vi "HexapodAcquireHardware.vi"(8 "error in (no error)":errorcluster, 11 "C-887 in":refnum<class "C-887.lvclass">) -> (0 "error out":errorcluster, 1 "Status Cluster":T1, 2 "In Motion":bool, 3 "C-887 out":refnum<class "C-887.lvclass">, 5 "Array":string[](array[string]))   [LabVIEW 2020, in "C-887.lvclass"]
uses:
  C-887.lvclass
  C:/GEECS/Developers Version/source/Device Drivers/HexapodPI/HexapodPI.lvclass
  HexapodPI.lvclass/HexapodPI.ctl
  C-887.lvclass/C-887.ctl
  subvis/activeChannel.ctl
  shared/OnOffTypeDef.ctl
  Read activeChannel.vi
  Read positioners.vi
  Read Settings.vi
  Write Status Cluster.vi
  Write activeChannel.vi
  Write Settings.vi
  shared/CompressAndUpdate(Poly)/CompressAndUpdate(Enum).vi
  shared/CompressAndUpdate(Poly)/CompressAndUpdate(Numeric).vi
  shared/CompressAndUpdate(Poly)/CompressAndUpdate(NumericArray).vi
  HexapodPI.lvclass
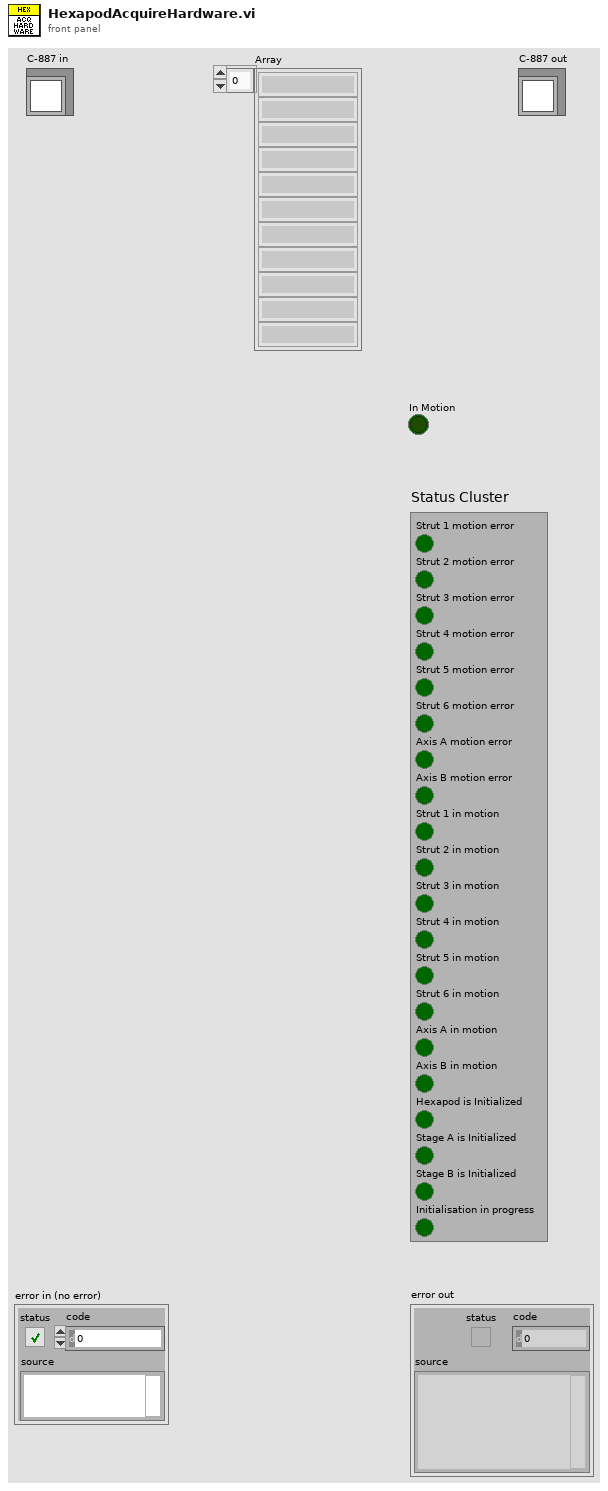
[diagram p1: front panel]
types:
  T1 = cluster{"Strut 1 motion error":bool, "Strut 2 motion error":bool, "Strut 3 motion error":bool, "Strut 4 motion error":bool, "Strut 5 motion error":bool, "Strut 6 motion error":bool, "Axis A motion error":bool, "Axis B motion error":bool, "Strut 1 in motion":bool, "Strut 2 in motion":bool, "Strut 3 in motion":bool, "Strut 4 in motion":bool, "Strut 5 in motion":bool, "Strut 6 in motion":bool, "Axis A in motion":bool, "Axis B in motion":bool, "Hexapod is Initialized":bool, "Stage A is Initialized":bool, "Stage B is Initialized":bool, "Initialisation in progress":bool}
  T2 = enum16{"Not referenced", "Homing", "Moving", "Ready"}
  T3 = typedef "activeChannel.ctl" = enum16{"xpos", "ypos", "zpos", "uangle", "vangle", "wangle", "n/a", "off"}
  T4 = typedef "HexapodPI.lvclass/settingHexapod_TypDEf.ctl" = cluster{"xpos":cluster{"Value":dbl, "Min":dbl, "Max":dbl, "StepSize":dbl, "Tolerance":dbl, "ValueActual":dbl}, "ypos":cluster{"Value":dbl, "Min":dbl, "Max":dbl, "StepSize":dbl, "Tolerance":dbl, "ValueActual":dbl}, "zpos":cluster{"Value":dbl, "Min":dbl, "Max":dbl, "StepSize":dbl, "Tolerance":dbl, "ValueActual":dbl}, "uangle":cluster{"Value":dbl, "Min":dbl, "Max":dbl, "StepSize":dbl, "Tolerance":dbl, "ValueActual":dbl}, "vangle":cluster{"Value":dbl, "Min":dbl, "Max":dbl, "StepSize":dbl, "Tolerance":dbl, "ValueActual":dbl}, "devaddress":string, "connectiontype":enum16{"TCPIP", "Serial"}, "hexinit":enum16{"Not referenced", "Referenced"}, "status":enum16{"Not referenced", "Homing", "Moving", "Ready"}, "relativeMove":cluster{"Zpos":T5, "Zneg":T5, "Xpos":T5, "Xneg":T5, "Ypos":T5, "Yneg":T5, "Wpos":T5, "Wneg":T5, "Vpos":T5, "Vneg":T5, "Upos":T5, "Uneg":T5}, "stepsize":cluster{"Value":dbl, "Min":dbl, "Max":dbl, "StepSize":dbl, "Tolerance":dbl, "ValueActual":dbl}, "LaserAxis":cluster{"u":dbl, "v":dbl, "w":dbl}, "PivotPoint":T6, "wangle":cluster{"Value":dbl, "Min":dbl, "Max":dbl, "StepSize":dbl, "Tolerance":dbl, "ValueActual":dbl}, "LaserAxes":T5, "speed":cluster{"Value":dbl, "Min":dbl, "Max":dbl, "StepSize":dbl, "Tolerance":dbl, "ValueActual":dbl}, "Simulation":T5, "xyzuvw":dbl[], "xyzuvw_tolerances":dbl[]}
  T5 = typedef "OnOffTypeDef.ctl" = enum16{"off", "on"}
  T6 = typedef "PivotPoint_TypDef.ctl" = cluster{"R":cluster{"Value":dbl, "Min":dbl, "Max":dbl, "StepSize":dbl, "Tolerance":dbl, "ValueActual":dbl}, "S":cluster{"Value":dbl, "Min":dbl, "Max":dbl, "StepSize":dbl, "Tolerance":dbl, "ValueActual":dbl}, "T":cluster{"Value":dbl, "Min":dbl, "Max":dbl, "StepSize":dbl, "Tolerance":dbl, "ValueActual":dbl}}
  T7 = cluster{"Zpos":T5, "Zneg":T5, "Xpos":T5, "Xneg":T5, "Ypos":T5, "Yneg":T5, "Wpos":T5, "Wneg":T5, "Vpos":T5, "Vneg":T5, "Upos":T5, "Uneg":T5}
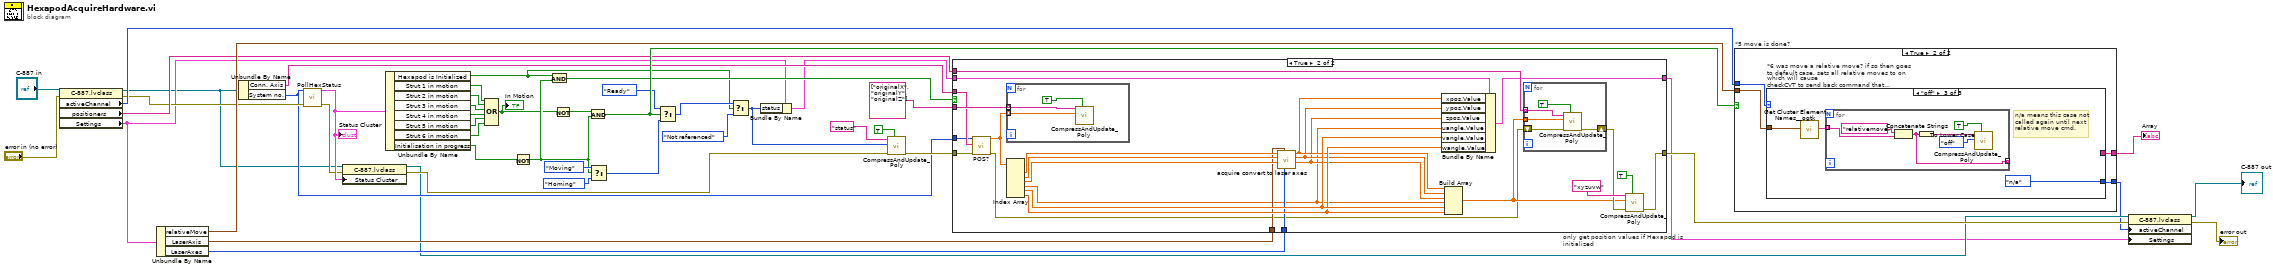
[diagram p0: block diagram]
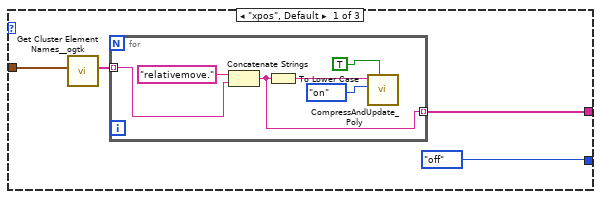
[diagram p3: hidden frame]
diagram:
  n1 = property class="C-887.lvclass"(reference="C-887 in", error in="error in (no error)") -> (reference out=w10:refnum<class "C-887.lvclass">, error out=w17:errorcluster, "activeChannel"=w21:T3, "positioners"=w19:string[], "Settings"=w12:T4)
  n2 = Unbundle By Name(w12) -> ("relativeMove"=w20:T7, "LaserAxis"=w22:cluster{"u":dbl, "v":dbl, "w":dbl}, "LaserAxes"=w23:T5)
  n3 = Unbundle By Name(w10) -> ("Conn. Axis"=w18:string[], "System no."=w13:i32)
  n4 = call "PollHexStatus.vi"("error in (no error)"=w17, "System no."=w13) -> ("error out"=w11:errorcluster, "Status Cluster 2"=w16:T1)  [unwired: 8 in]
  "Status Cluster" <- w16
  n5 = property class="C-887.lvclass"(reference=w10, error in=w11, "Status Cluster"=w16) -> (reference out=w5:refnum<class "C-887.lvclass">, error out=w9:errorcluster)
  n6 = Unbundle By Name(w16) -> ("Hexapod is Initialized"=w7:bool, "Strut 1 in motion"=w33:bool, "Strut 2 in motion"=w28:bool, "Strut 3 in motion"=w29:bool, "Strut 4 in motion"=w30:bool, "Strut 5 in motion"=w31:bool, "Strut 6 in motion"=w32:bool, "Initialisation in progress"=w27:bool)
  n7 = Compound Arithmetic op=OR(w33, w28, w29, w30, w31, w32) -> (w36:bool)
  "In Motion" <- w36
  n8 = Not(x=w27) -> (.not. x?=w37:bool)
  n9 = And(x=w7, y=w37) -> (x .and. y?=w34:bool)
  n10 = Not(x=w36) -> (.not. x?=w45:bool)
  n11 = And(x=w45, y=w37) -> (x .and. y?=w46:bool)
  n12 = Select(t=T2."Moving" ("Settings.status"), s=w37, f=T2."Homing" ("Settings.status")) -> (s? t:f=w38:T2)
  n13 = Select(t=T2."Ready" ("Settings.status"), s=w46, f=w38) -> (s? t:f=w41:T2)
  n14 = Select(t=w41, s=w7, f=T2."Not referenced" ("Settings.status")) -> (s? t:f=w15:T2)
  n15 = Bundle By Name(cluster=w12, "status"=w15) -> (w8:T4)
  n16 = call-poly "CompressAndUpdate_Poly.vi"("force CVT update (false)"=TRUE, "error in"=w9, "enum variant"=w15, "command or variable name"="status") -> ("error out"=w14:errorcluster)  [unwired: 7 in]
  n17 = case "only get position values if Hexapod is initialized" shown="True" w34 {
    tunnel: [w49 w61] -> w6
    tunnel: w14 -> [w49 w59]
    tunnel: w19 -> [_ w74]
    tunnel: w18 -> [_ w58]
    tunnel: string[] ["originalX", "originalY", "originalZ"] -> [_ w68]
    tunnel: w22 -> [_ w66]
    tunnel: w23 -> [_ w65]
    tunnel: w13 -> [_ w57]
    tunnel: w8 -> [w48 w54]
    tunnel: [w48 w53] -> w2
    frame False {
    }
    frame True {
      n18 = call "POS?.vi"("System no."=w57, "Axes to query"=w58, "error in"=w59) -> ("Position"=w56:dbl[], "error out"=w55:errorcluster)  [unwired: 15 in]
      n19 = for {
        tunnel: w56 -> [w76] mode=indexing
        tunnel: w68 -> [w75] mode=indexing
        n20 = call-poly "CompressAndUpdate_Poly.vi"("force CVT update (false)"=TRUE, "Numeric"=w76, "command or variable name"=w75) -> ()  [unwired: 8 in, 1 out]
      }
      n21 = Index Array(array=w56) -> (element #1=w73:dbl, element #2=w72:dbl, element #3=w71:dbl, element #4=w50:dbl, element #5=w70:dbl, element #6=w69:dbl)  [unwired: 6 in]
      n22 = call "acquire convert to laser axes.vi"("Settings.Trigger"=w65, "LaserAxis"=w66, "z in"=w71, "y in"=w72, "x in"=w73) -> ("z out"=w51:dbl, "y out"=w52:dbl, "x out"=w67:dbl)  [unwired: 4 in]
      n23 = Bundle By Name(cluster=w54, "xpos.Value"=w67, "ypos.Value"=w52, "zpos.Value"=w51, "uangle.Value"=w50, "vangle.Value"=w70, "wangle.Value"=w69) -> (w53:T4)
      n24 = Build Array(w67, w52, w51, w50, w70, w69) -> (w60:dbl[])
      n25 = for {
        tunnel: w60 -> [w79] mode=indexing
        tunnel: w74 -> [w78] mode=indexing
        shift-right: [w82] -> w62
        shift-left: w55 -> [w80]
        n26 = call-poly "CompressAndUpdate_Poly.vi"("force CVT update (false)"=TRUE, "error in"=w80, "Numeric"=w79, "command or variable name"=w78) -> ("error out"=w82:errorcluster)  [unwired: 7 in]
      }
      n27 = call-poly "CompressAndUpdate_Poly.vi"("force CVT update (false)"=TRUE, "error in"=w62, "Numeric Array"=w60, "command or variable name"="xyzuvw") -> ("error out"=w61:errorcluster)  [unwired: 7 in]
    }
  }
  n28 = case "*5 move is done?" shown="True" w46 {
    tunnel: w20 -> [_ w86]
    tunnel: w21 -> [_ w85]
    tunnel: [_ w84] -> w26
    tunnel: [_ w83] -> w1
    frame False {
    }
    frame True {
      n29 = case "*6 was move a relative move? if so then goes to default case. sets all relative moves to on which will cause\ncheckCVT to send back command that setrelative move was done. sets activechannel to off so next acquire will\nset all relative move enums to off." shown="\"off\"" w85 {
        tunnel: w86 -> [w90 _ w98]
        tunnel: [w88 _ _] -> w84
        tunnel: [activeChannel."off" ("activeChannel") _ activeChannel."n/a" ("activeChannel")] -> w83
        frame "xpos", Default {
          n30 = call <userlib>:"Get Cluster Element Names__ogtk.vi"("Cluster"=w90) -> ("Element Names"=w89:string[])  [unwired: 9 in, 1 out]
          n31 = for {
            tunnel: w89 -> [w96] mode=indexing
            tunnel: [w92] -> w88 mode=indexing
            n32 = Concatenate Strings("relativemove." ("string"), w96) -> (w92:string)
            n33 = To Lower Case(string=w92) -> (all lower case string=w91:string)
            n34 = call-poly "CompressAndUpdate_Poly.vi"("force CVT update (false)"=TRUE, "enum variant"=OnOffTypeDef."on" ("Zpos"), "command or variable name"=w91) -> ()  [unwired: 8 in, 1 out]
          }
        }
        frame "n/a" {
        }
        frame "off" {
          # "n/a means this case not\ncalled again until next\nrelative move cmd."
          n35 = call <userlib>:"Get Cluster Element Names__ogtk.vi"("Cluster"=w98) -> ("Element Names"=w99:string[])  [unwired: 9 in, 1 out]
          n36 = for {
            tunnel: w99 -> [w105] mode=indexing
            tunnel: [w101] -> _ mode=indexing
            n37 = Concatenate Strings("relativemove." ("string"), w105) -> (w101:string)
            n38 = To Lower Case(string=w101) -> (all lower case string=w100:string)
            n39 = call-poly "CompressAndUpdate_Poly.vi"("force CVT update (false)"=TRUE, "enum variant"=OnOffTypeDef."off" ("Zpos"), "command or variable name"=w100) -> ()  [unwired: 8 in, 1 out]
          }
        }
      }
    }
  }
  "Array" <- w26
  n40 = property class="C-887.lvclass"(reference=w5, error in=w6, "activeChannel"=w1, "Settings"=w2) -> (reference out=→"C-887 out":refnum<class "C-887.lvclass">, error out=→"error out":errorcluster)
